vi "Check3DPointInsideBox.vi"(10 "3D Cuboid":T1, 11 "3D Point":T2) -> (3 "PointIsInsideCuboid":bool)   [LabVIEW 2023]
uses:
  3Dpoint.ctl
  3DCuboid.ctl
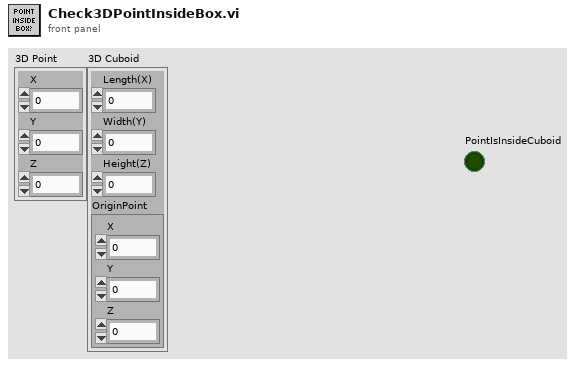
[diagram p1: front panel]
types:
  T1 = typedef "3DCuboid.ctl" = cluster{"Length(X)":dbl, "Width(Y)":dbl, "Height(Z)":dbl, "OriginPoint":T2}
  T2 = typedef "3Dpoint.ctl" = cluster{"X":dbl, "Y":dbl, "Z":dbl}
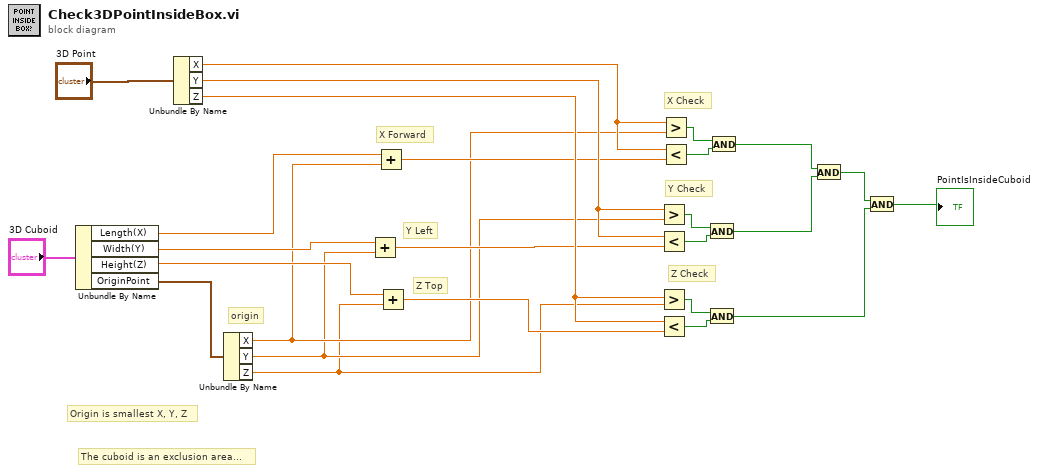
[diagram p0: block diagram]
diagram:
  # "The cuboid is an exclusion area..."
  # "origin"
  # "Origin is smallest X, Y, Z"
  # "X Check"
  # "Y Check"
  # "Z Check"
  # "Z Top"
  # "Y Left"
  # "X Forward"
  n1 = Unbundle By Name("3D Cuboid") -> ("Length(X)"=w24:dbl, "Width(Y)"=w22:dbl, "Height(Z)"=w23:dbl, "OriginPoint"=w6:T2)
  n2 = Unbundle By Name("3D Point") -> ("X"=w10:dbl, "Y"=w9:dbl, "Z"=w8:dbl)
  n3 = Unbundle By Name(w6) -> ("X"=w3:dbl, "Y"=w2:dbl, "Z"=w1:dbl)
  n4 = Add(x=w22, y=w2) -> (x+y=w5:dbl)
  n5 = Add(x=w24, y=w3) -> (x+y=w7:dbl)
  n6 = Add(x=w23, y=w1) -> (x+y=w4:dbl)
  n7 = Greater?(x=w9, y=w2) -> (0:w17:bool)
  n8 = Less?(x=w9, y=w5) -> (x < y?=w16:bool)
  n9 = Greater?(x=w8, y=w1) -> (0:w15:bool)
  n10 = Less?(x=w8, y=w4) -> (x < y?=w14:bool)
  n11 = Greater?(x=w10, y=w3) -> (0:w21:bool)
  n12 = Less?(x=w10, y=w7) -> (x < y?=w20:bool)
  n13 = And(x=w17, y=w16) -> (x .and. y?=w12:bool)
  n14 = And(x=w15, y=w14) -> (x .and. y?=w13:bool)
  n15 = And(x=w21, y=w20) -> (x .and. y?=w11:bool)
  n16 = And(x=w11, y=w12) -> (x .and. y?=w18:bool)
  n17 = And(x=w18, y=w13) -> (x .and. y?=→"PointIsInsideCuboid":bool)
